vi "DHE_DRV_set_num_reads.vi"(0 "fd":i32, 5 "num_reads":i32=1, 11 "error in (no error)":errorcluster) -> (4 "fd out":i32, 8 "return value":i32, 15 "error out":errorcluster)   [LabVIEW 2016]
doc: "This VI closes the I/O interface with the instrument."
uses:
  c/lib/libarcDHE.so
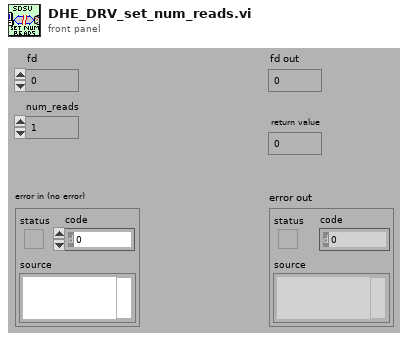
[diagram p1: front panel]
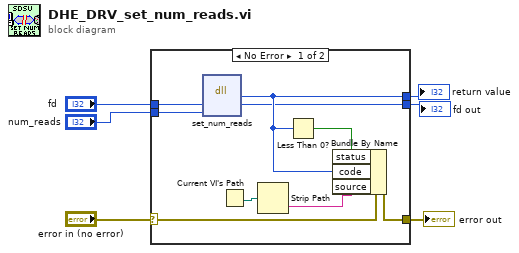
[diagram p0: block diagram]
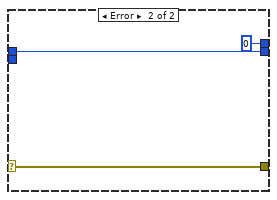
[diagram p2: hidden frame]
diagram:
  n1 = case shown="No Error" "error in (no error)" {
    selector: "error in (no error)" -> [w7 w16]
    tunnel: "fd" -> [w15 w18]
    tunnel: [w13 0] -> w5
    tunnel: [w10 w16] -> w4
    tunnel: "num_reads" -> [w9 _]
    tunnel: [w8 w18] -> w2
    frame No Error {
      n2 = dll-call lib="home/simager/panview/PAN/Modules/SDSU/private/c/lib/libarcDHE.so" fn="set_num_reads"("fd"=w15, "num_reads"=w9) -> (w13:i32, "fd"=w8:i32)  [unwired: 4 in, 2 out]
      n3 = Current VI's Path() -> (path=w12:path)
      n4 = Strip Path(path=w12) -> (name=w11:string)  [unwired: 1 out]
      n5 = Less Than 0?(x=w13) -> (x < 0?=w14:bool)
      n6 = Bundle By Name(cluster=w7, "status"=w14, "code"=w13, "source"=w11) -> (w10:errorcluster)
    }
    frame Error {
    }
  }
  "error out" <- w4
  "return value" <- w5
  "fd out" <- w2
